vi "CheckPrepareShot.vi"(8 "error in (no error)":errorcluster, 10 "Game":refnum<class "Game.lvclass">, 11 "object in":refnum<class "PrimaryAttackerRole.lvclass">) -> (0 "error out":errorcluster, 1 "nextState":T2, 2 "tactic":T1, 3 "object out":refnum<class "PrimaryAttackerRole.lvclass">)   [LabVIEW 2023, in "PrimaryAttackerRole.lvclass"]
uses:
  PrimaryAttackerRole.lvclass
  PrimaryAttackerRole_states.ctl
  Robot_class/tactics.ctl
  Game_class/Game.lvclass
  PrimaryAttackerRole.lvclass/PrimaryAttackerRole.ctl
panel:
  in  "prepareTime":dbl=0.5
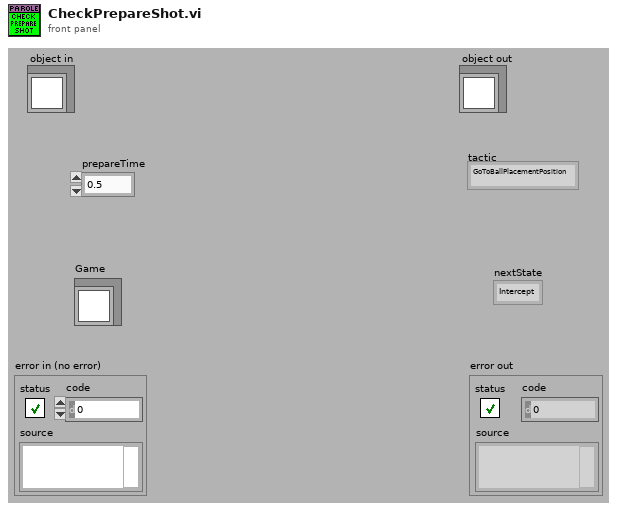
[diagram p1: front panel]
types:
  T1 = typedef "tactics.ctl" = enum16{"GoToBallPlacementPosition", "PlaceBall", "GoToBallPlacement", "5Robots", "BallPlacementEnemy", "ReceivePassInFuturePoint", "Roller", "PrepareRollToPassRollerGoTo", "PrepareRollToPassReceiverGoTo", "WaitRoll", "PositionToRoll", "PenaltyAttacker", "PassObserver", "PenaltyDefense", "TableReceiverTactic", "Test", "DefendGoal", "Marker", "FollowAttacker", "DefendArea", "Shoot", "AttackerAimGoal", "AttackerBallOutOfField", "AttackerBlock", "AttackerStop", "Duelist", "Halt", "ZigZag", "GoTo", "Timeout", "KickToBestRobot", "KickToPassReceiver", "PositionToReceivePass", "WaitPass", "Position", "Intercept", "PrepareShot", "Pass"}
  T2 = typedef "PrimaryAttackerRole.lvclass/PrimaryAttackerRole_states.ctl" = enum16{"Intercept", "PrepareShot", "Shoot", "Pass"}
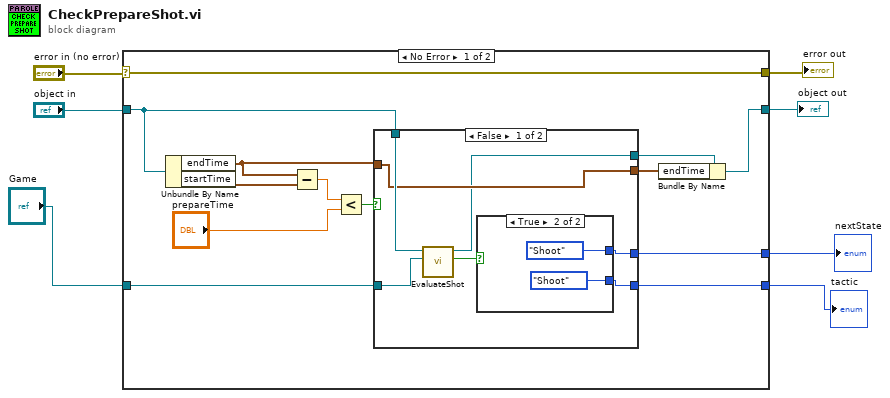
[diagram p0: block diagram]
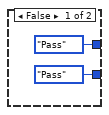
[diagram p2: hidden frame]
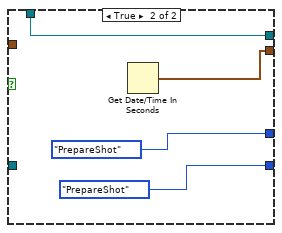
[diagram p3: hidden frame]
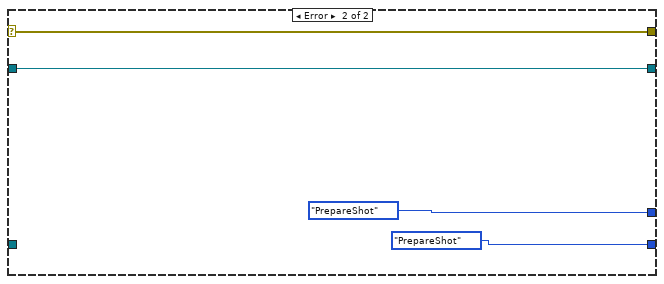
[diagram p4: hidden frame]
diagram:
  n1 = case shown="No Error" "error in (no error)" {
    selector: "error in (no error)" -> [w20 w39]
    tunnel: [w20 w39] -> w6
    tunnel: [w19 w38] -> w4
    tunnel: "object in" -> [w10 w38]
    tunnel: [w12 PrimaryAttackerRole_states."PrepareShot" ("nextState")] -> w3
    tunnel: [w11 tactics."PrepareShot" ("tactic")] -> w2
    tunnel: "Game" -> [w9 _]
    frame No Error {
      n2 = Unbundle By Name(w10) -> ("endTime"=w13:timestamp, "startTime"=w18:timestamp)
      n3 = Subtract(x=w13, y=w18) -> (x-y=w17:dbl)
      n4 = Less?(x=w17, y="prepareTime") -> (x < y?=w15:bool)
      n5 = case shown="False" w15 {
        tunnel: [w23 w33] -> w14
        tunnel: w13 -> [w23 _]
        tunnel: [w27 PrimaryAttackerRole_states."PrepareShot" ("nextState")] -> w12
        tunnel: [w26 tactics."PrepareShot" ("tactic")] -> w11
        tunnel: w10 -> [w25 w32]
        tunnel: w9 -> [w24 _]
        tunnel: [w21 w32] -> w8
        frame False {
          n6 = call "EvaluateShot.vi"("Game"=w24, "object in"=w25) -> ("Shoot"=w22:bool, "object out"=w21:refnum<class "PrimaryAttackerRole.lvclass">)  [unwired: 7 in, 1 out]
          n7 = case shown="True" w22 {
            tunnel: [PrimaryAttackerRole_states."Pass" ("nextState") PrimaryAttackerRole_states."Shoot" ("nextState")] -> w27
            tunnel: [tactics."Pass" ("tactic") tactics."Shoot" ("tactic")] -> w26
            frame False {
            }
            frame True {
            }
          }
        }
        frame True {
          n8 = Get Date/Time In Seconds() -> (seconds since 1Jan1904=w33:timestamp)
        }
      }
      n9 = Bundle By Name(cluster=w8, "endTime"=w14) -> (w19:refnum<class "PrimaryAttackerRole.lvclass">)
    }
    frame Error {
    }
  }
  "error out" <- w6
  "object out" <- w4
  "nextState" <- w3
  "tactic" <- w2
